vi "ex_InterleaveColHdngs.vi"(6 "empty duplicate tokens (T)":bool=TRUE, 7 "channels":i32, 8 "col heading tokens":string[](array[string]), 9 "col heading data":string[][](table)) -> (3 "modified heading data":string[][](table))   [LabVIEW 2017]
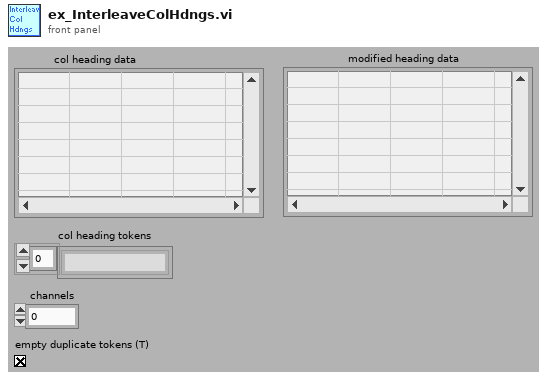
[diagram p1: front panel]
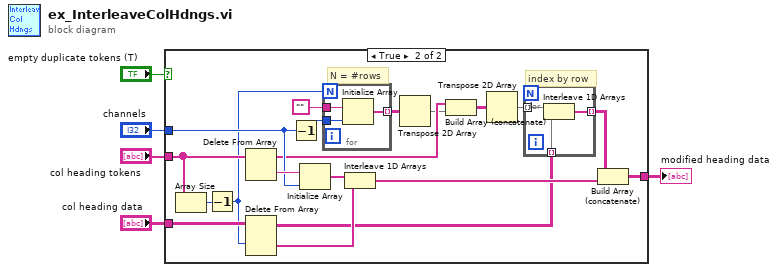
[diagram p0: block diagram]
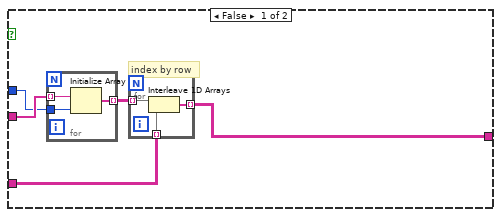
[diagram p2: hidden frame]
diagram:
  n1 = case shown="True" "empty duplicate tokens (T)" {
    tunnel: "col heading tokens" -> [w10 w33]
    tunnel: "col heading data" -> [w8 w34]
    tunnel: [w6 w30] -> w3
    tunnel: "channels" -> [w7 w23]
    frame False {
      # "index by row"
      n2 = for {
        tunnel: [w12] -> w9 mode=indexing
        tunnel: w10 -> [w13] mode=indexing
        tunnel: w7 -> [w11]
        n3 = Initialize Array(w13, w11) -> (w12:string[])
      }
      n4 = for {
        tunnel: w9 -> [w16] mode=indexing
        tunnel: w8 -> [w15] mode=indexing
        tunnel: [w14] -> w6 mode=indexing
        n5 = Interleave 1D Arrays(w16, w15) -> (w14:string[])
      }
    }
    frame True {
      # "index by row"
      # "N = #rows"
      n6 = Array Size(array=w33) -> (size(s)=w18:i32)
      n7 = Decrement(x=w18) -> (x-1=w17:i32)
      n8 = Delete From Array(array=w33) -> (deleted portion=w32:string, array with subset deleted=w21:string[])  [unwired: 2 in]
      n9 = Delete From Array(array=w34, index (row)=w17) -> (deleted portion=w31:string[], array with subset deleted=w27:string[][])  [unwired: 2 in]
      n10 = Decrement(x=w23) -> (x-1=w25:i32)
      n11 = Initialize Array(w32, w23) -> (w35:string[])
      n12 = for {
        N: w17 -> [_]
        tunnel: [w41] -> w24 mode=indexing
        tunnel: "" -> [w40]
        tunnel: w25 -> [w39]
        n13 = Initialize Array(w40, w39) -> (w41:string[])
      }
      n14 = Interleave 1D Arrays(w35, w31) -> (w29:string[])
      n15 = Transpose 2D Array(2D array=w24) -> (transposed array=w20:string[][])
      n16 = Build Array (concatenate)(w21, w20) -> (w22:string[][])
      n17 = Transpose 2D Array(2D array=w22) -> (transposed array=w19:string[][])
      n18 = for {
        tunnel: w19 -> [w38] mode=indexing
        tunnel: [w37] -> w28 mode=indexing
        tunnel: w27 -> [w36] mode=indexing
        n19 = Interleave 1D Arrays(w38, w36) -> (w37:string[])
      }
      n20 = Build Array (concatenate)(w28, w29) -> (w30:string[][])
    }
  }
  "modified heading data" <- w3
